vi "Send.vi"(8 "error in":errorcluster, 11 "Data":string="Send") -> (0 "error out":errorcluster)   [LabVIEW 2016, in "TCP.lvlib"]
uses:
  TCP.lvlib
  Support/Message Queue/Enqueue Message (Single).vi
  support/Message Queue/Message Queue.lvlib
panel:
  in  "Action":enum16{"GET", "SET"}(ring)
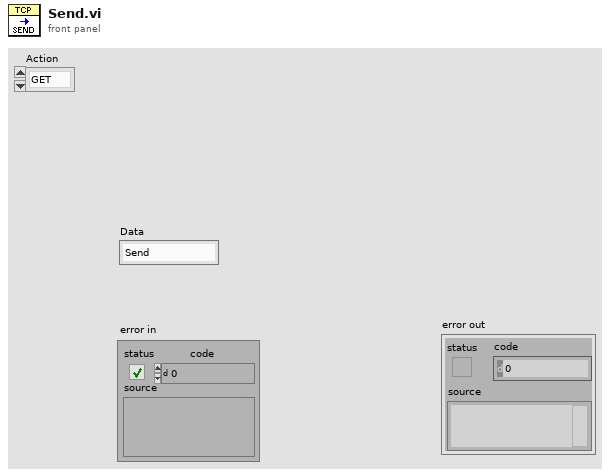
[diagram p1: front panel]
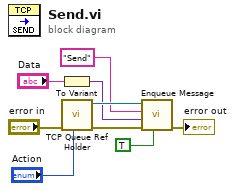
[diagram p0: block diagram]
diagram:
  n1 = To Variant(anything="Data") -> (Variant=w4:variant)
  n2 = call "TCP Queue Ref Holder.vi"("Action"="Action", "error in"="error in") -> ("error out"=w8:errorcluster, "Input Message Queue"=w6:refnum<queue>)  [unwired: 8 in]
  n3 = call-poly "Enqueue Message.vi"("Priority Message? (F)"=TRUE, "error in (no error)"=w8, "Message Data"=w4, "Message"="Send", "Message Queue"=w6) -> ("error out"=→"error out":errorcluster)  [unwired: 5 in, 1 out]
